vi "collect pulses.vi"(8 "error in (no error)":errorcluster, 9 "max number of pulses to show":dbl, 10 "time range":cluster{dbl, dbl}(slide)={9.216589861751153, 78525345.62211981} scale=0.0..50.0 scale format="%#_6p sec", 11 "pulse_gen_and_detect_p2p in":refnum<class "pulse_gen_and_detect_p2p.lvclass">) -> (0 "error out":errorcluster, 2 "PDW":cluster{"PDW":T1[], "Ton":dbl[]} {"PDW"."frequency shift" format="%#_12f"}, 3 "pulse_gen_and_detect_p2p out":refnum<class "pulse_gen_and_detect_p2p.lvclass">)   [LabVIEW 2021, in "pulse_gen_and_detect_p2p.lvclass"]
uses:
  pulse_gen_and_detect_p2p.lvclass
  pulse_tx_vis/pdw.ctl
  pulse_tx_vis/CTL/mode_type.ctl
  fpga/vis/pulse detector/PDW interpoter params.ctl
  pulse_gen_and_detect_p2p.lvclass/pulse_gen_and_detect_p2p.ctl
  <instrlib>/_niInstr/Basic Elements/v1/FPGA/Private/Count Up U64.vi
  device_type/device_type.lvclass
  <instrlib>/_niInstr/Basic Elements/v1/FPGA/niInstr Basic Elements v1 FPGA.lvlib
panel:
  out "error out 2":errorcluster
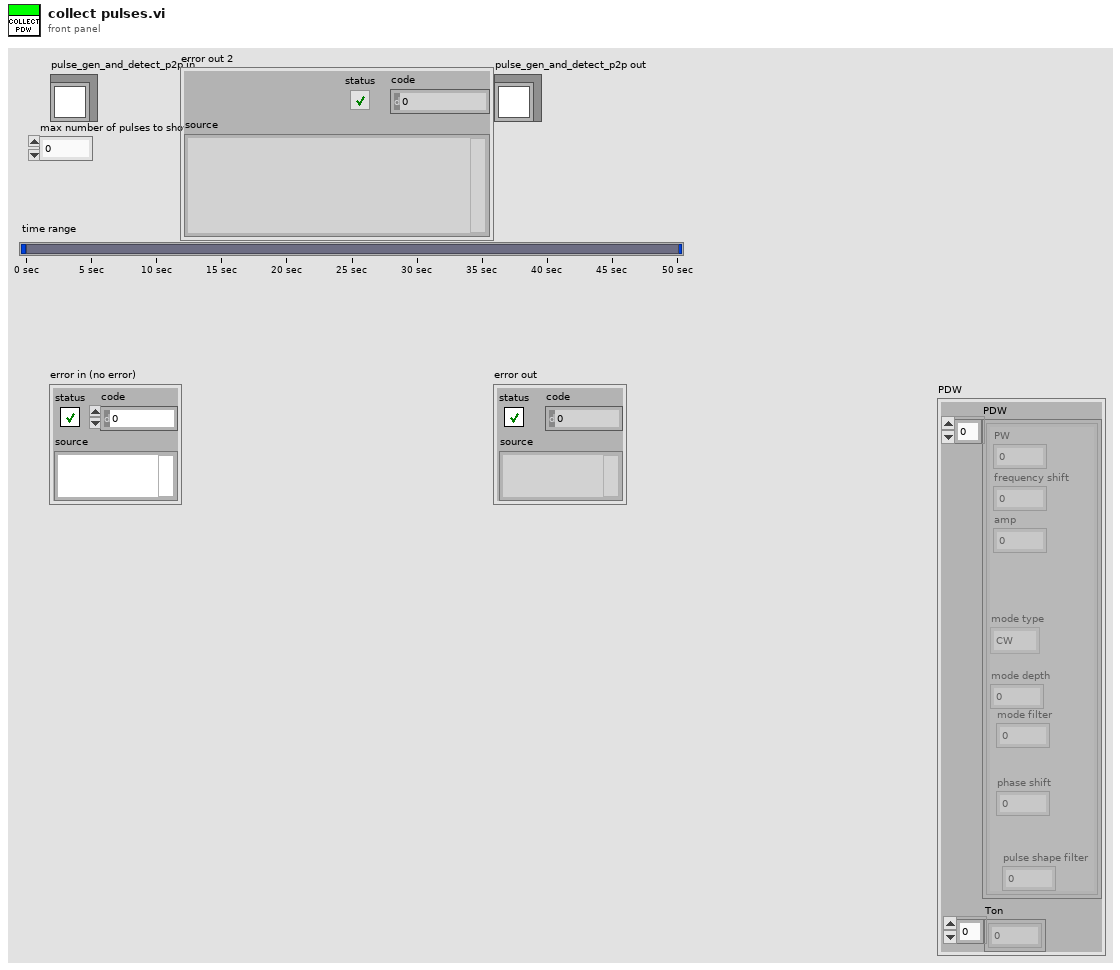
[diagram p1: front panel]
types:
  T1 = typedef "pdw.ctl" = cluster{"PW":u32, "frequency shift":fxp<+/-,48,0>, "amp":fxp<+/-,18,1>, "mode type":T2, "mode depth":u32, "mode filter":u8, "phase shift":fxp<+/-,16,1>, "pulse shape filter":u8}
  T2 = typedef "mode_type.ctl" = enum8{"CW", "NC - CW", "NC - cw", "LFM", "BPSK", "QPSK"}
  T3 = typedef "PDW interpoter params.ctl" = cluster{"Fs (Hz)":dbl, "fft size ":u32, "F base (Hz)":dbl, "min AMP (dB)":dbl, "PW low bar (fft cycle)":dbl, "Pw high bar (fft cycle)":dbl, "lo likege removal (fft bin)":i32, "max gap (fft cycle)":dbl}
  T4 = enum16{"open", "open or create", "create or replace", "create", "open (read-only)"}
  T5 = cluster{"min PW (fft cycels)":u16, "max PW (fft cycels)":u16, "max gap (fft cycels)":u8, "detection bar (liniar amp)":fxp<+,64,63>, "peak detect":bool}
  T6 = cluster{"f":dbl, "pw":dbl, "amp":dbl, "tend":dbl}[]
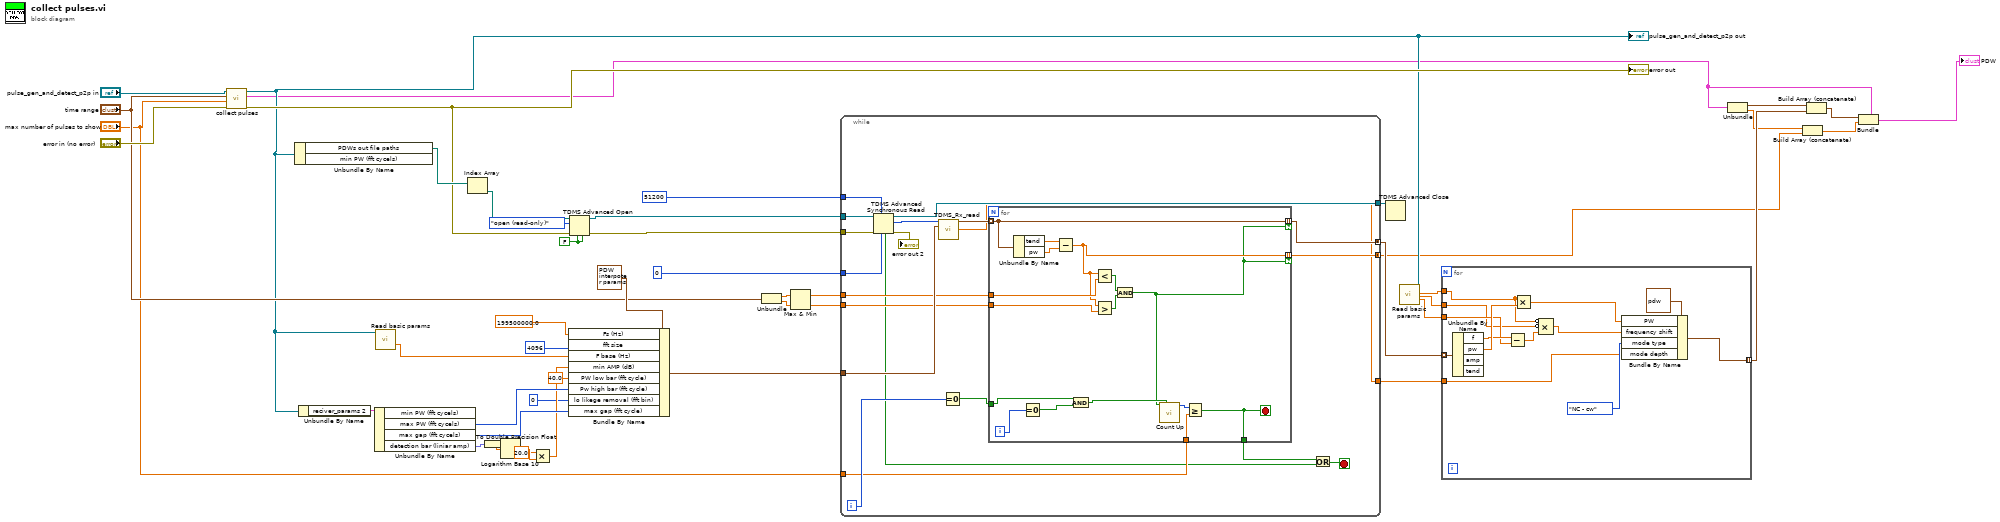
[diagram p0: block diagram]
diagram:
  w2 = FALSE ("enable asynchronous? (T)")
  n1 = call-parent "collect pulses.vi"("error in (no error)"="error in (no error)", "max number of pulses to show"="max number of pulses to show", "time range"="time range", "device_type in"="pulse_gen_and_detect_p2p in") -> ("error out"=w42:errorcluster, "PDW"=w5:cluster{"PDW":T1[], "Ton":dbl[]}, "device_type out"=w17:refnum<class "pulse_gen_and_detect_p2p.lvclass">)  [unwired: 5 in]
  "error out" <- w42
  "pulse_gen_and_detect_p2p out" <- w17
  n2 = Unbundle By Name(w17) -> ("PDWs out file paths"=w45:path[])  [unwired: 1 out]
  n3 = Unbundle By Name(w17) -> ("reciver_params 2"=w34:T5)
  n4 = Unbundle By Name(w34) -> ("max PW (fft cycels)"=w32:u16, "max gap (fft cycels)"=w33:u8, "detection bar (liniar amp)"=w31:fxp<+,64,63>)  [unwired: 1 out]
  n5 = call-dynamic "Read basic params.vi"("device_type in"=w17) -> ("center frequency (Hz)"=w26:dbl)  [unwired: 13 in, 5 out]
  n6 = Index Array(array=w45) -> (element=w44:path)  [unwired: 1 in]
  n7 = To Double Precision Float(number=w31) -> (double precision float=w30:dbl)
  n8 = Logarithm Base 10(1:w30) -> (0:w29:dbl)
  n9 = Multiply(x=20.0, y=w29) -> (x*y=w27:dbl)
  n10 = Bundle By Name(cluster=T3 {"Fs (Hz)"=200000000.0, "fft size "=4096, "F base (Hz)"=5000000000.0, "min AMP (dB)"=60.0, "PW low bar (fft cycle)"=6.0, "Pw high bar (fft cycle)"=500000000000.0, "lo likege removal (fft bin)"=10, "max gap (fft cycle)"=1.0} ("PDW interpoter params"), "Fs (Hz)"=199500000.0, "fft size"=u32 4096, "F base (Hz)"=w26, "min AMP (dB)"=w27, "PW low bar (fft cycle)"=40.0, "Pw high bar (fft cycle)"=w32, "lo likege removal (fft bin)"=0, "max gap (fft cycle)"=w33) -> (w36:T3)
  n11 = TDMS Advanced Open(4:w2, 6:w2, 8:w42, 10:T4."open (read-only)" ("operation (0:open)"), 11:w44) -> (0:w40:errorcluster, 3:w41:refnum<k34>)  [unwired: 1 out]
  n12 = Unbundle("time range") -> (w22:dbl, w23:dbl)
  n13 = Max & Min(x=w22, y=w23) -> (max(x,y)=w19:dbl, min(x,y)=w20:dbl)
  n14 = while {
    tunnel: w41 -> [w67]
    tunnel: w40 -> [w66]
    tunnel: u64 0 -> [w65]
    tunnel: i64 51200 ("count (-1)") -> [w64]
    tunnel: w36 -> [w62]
    tunnel: [w60] -> w24
    tunnel: w20 -> [w59]
    tunnel: w19 -> [w58]
    tunnel: "max number of pulses to show" -> [w55]
    tunnel: [w51] -> w16 mode=concatenating
    tunnel: [w50] -> w8 mode=concatenating
    tunnel: [w49] -> w12
    i -> [w57]
    stop <- w52 stop-if-true
    n15 = TDMS Advanced Synchronous Read(6:w65, 7:w64, 8:w66, 11:w67) -> (0:→"error out 2":errorcluster, 2:w63:u64[], 3:w60:refnum<k34>, 4:w54:bool)
    n16 = call "TDMS_Rx_read.vi"("Array in"=w63, "PDW interpoter params"=w62) -> ("Array"=w61:T6, "frequncy resolotion"=w49:dbl)  [unwired: 11 in, 1 out]
    n17 = Equal To 0?(x=w57) -> (x = 0?=w56:bool)
    n18 = for {
      tunnel: w61 -> [w70] mode=indexing
      tunnel: w59 -> [w80]
      tunnel: w58 -> [w79]
      tunnel: w56 -> [w76]
      tunnel: w55 -> [w73]
      tunnel: [w71] -> w53
      tunnel: [w70] -> w51 mode=indexing if=w68
      tunnel: [w69] -> w50 mode=indexing if=w68
      i -> [w77]
      stop <- w71 stop-if-true
      n19 = Unbundle By Name(w70) -> ("tend"=w83:dbl, "pw"=w82:dbl)
      n20 = Equal To 0?(x=w77) -> (x = 0?=w78:bool)
      n21 = Subtract(x=w83, y=w82) -> (x-y=w69:dbl)
      n22 = And(x=w76, y=w78) -> (x .and. y?=w74:bool)
      n23 = Less?(x=w69, y=w79) -> (x < y?=w72:bool)
      n24 = Greater?(x=w69, y=w80) -> (0:w81:bool)
      n25 = And(x=w72, y=w81) -> (x .and. y?=w68:bool)
      n26 = call-poly <instrlib>:"Count Up.vi"("increment"=w68, "reset"=w74) -> ("count out"=w75:u64)  [unwired: 13 in]
      n27 = Greater Or Equal?(x=w75, y=w73) -> (x >= y?=w71:bool)
    }
    n28 = Or(x=w53, y=w54) -> (x .or. y?=w52:bool)
  }
  n29 = TDMS Advanced Close(11:w24) -> ()  [unwired: 3 in, 2 out]
  n30 = call-dynamic "Read basic params.vi"("device_type in"=w17) -> ("Fs  FPGA"=w15:dbl, "SPC"=w13:dbl, "center frequency (Hz)"=w14:dbl)  [unwired: 13 in, 3 out]
  n31 = for {
    tunnel: w16 -> [w94] mode=indexing
    tunnel: w15 -> [w87]
    tunnel: w14 -> [w90]
    tunnel: w13 -> [w88]
    tunnel: w12 -> [w85]
    tunnel: [w84] -> w11 mode=indexing
    n32 = Unbundle By Name(w94) -> ("f"=w91:dbl, "pw"=w93:dbl)  [unwired: 2 out]
    n33 = Subtract(x=w91, y=w90) -> (x-y=w89:dbl)
    n34 = Multiply(x=w87, y=w93) -> (x*y=w92:dbl)
    n35 = Compound Arithmetic op=MULTIPLY(invert w87, invert w88, w89) -> (w86:dbl)
    n36 = Bundle By Name(cluster=T1 {"PW"=0, "frequency shift"=0.0, "amp"=0.0, "mode type"=enum."CW", "mode depth"=0, "mode filter"=0, "phase shift"=0.0, "pulse shape filter"=0} ("Cluster"), "PW"=w92, "frequency shift"=w86, "mode type"=mode_type."NC - cw", "mode depth"=w85) -> (w84:T1)
  }
  n37 = Unbundle(w5) -> ("PDW"=w10:T1[], "Ton"=w9:dbl[])
  n38 = Build Array (concatenate)(w9, w8) -> (w6:dbl[])
  n39 = Build Array (concatenate)(w10, w11) -> (w7:T1[])
  n40 = Bundle(cluster=w5, "PDW"=w7, "Ton"=w6) -> (→"PDW":cluster{"PDW":T1[], "Ton":dbl[]})
